vi "SetMatlabBoundControlCollectionVariant.vi"(10 "BoundControlCollectionVariant in":variant, 11 "ExpID":string) -> (3 "BoundControlCollectionVariant":variant)   [LabVIEW 2017]
uses:
  MatlabGlobals.vi
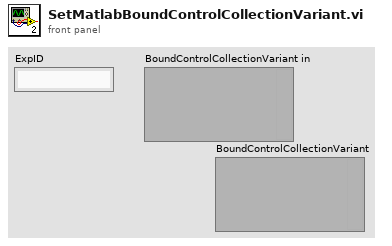
[diagram p1: front panel]
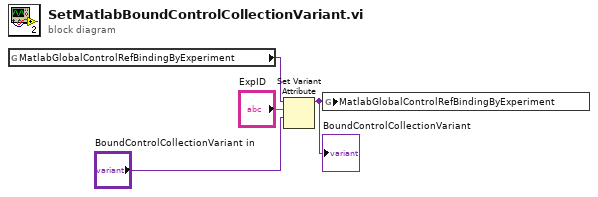
[diagram p0: block diagram]
diagram:
  n1 = global read "MatlabGlobals.vi" "MatlabGlobalControlRefBindingByExperiment"() -> (w4:variant)
  n2 = Set Variant Attribute(Variant=w4, name="ExpID", value="BoundControlCollectionVariant in") -> (Variant out=w1:variant)  [unwired: 1 in, 2 out]
  "BoundControlCollectionVariant" <- w1
  n3 = global write "MatlabGlobals.vi" "MatlabGlobalControlRefBindingByExperiment"(w1) -> ()
